vi "rsidr_core_global.vi"() -> ()   [LabVIEW 2015, in "Rohde&Schwarz CMXP GPRF.lvlib"] (continued)
"Read Callback"="", "Write Callback"="", "Supported Models"="", "Instrument Options"="", "Flags"=0, "Help"=""}, {"Level"=3, "Class Only"=FALSE, "Identifier"="RSCMXPGPRF_ATTR_GENERATOR_OUTPUT_CONNECTOR", "Descriptive Name"="Generator Output Connector", "Data Type"=0, "Command"="ROUT:GPRF:GEN{instance}:RFS:CONN", "Access"=2, "Range Table"="rsCmxpGprf_rngOutputConnector", "Read Callback"="", "Write Callback"="", "Supported Models"="", "Instrument Options"="", "Flags"=0, "Help"="Selects the output connector for the RF generator signal.\n\nAvailable Repeated Capabilities:\ninstance: i0, i1, i2, i3, i4, i5, i6, i7, i8, i9, i10, i11, i12, i13, i14, i15, i16, i17, i18, i19, i20, i21, i22, i23, i24, i25, i26, i27, i28, i29, i30, i31, i32\r\n\nRemote-control command(s):\nROUTe:GPRF:GEN<i>:RFSettings:CONNector"}, {"Level"=3, "Class Only"=FALSE, "Identifier"="RSCMXPGPRF_ATTR_GENERATOR_EXTERNAL_ATTENUTATION", "Descriptive Name"="Generator External Attenutation", "Data Type"=1, "Command"="SOUR:GPRF:GEN{instance}:RFS:EATT", "Access"=2, "Range Table"="rsCmxpGprf_rngExtAtt", "Read Callback"="", "Write Callback"="", "Supported Models"="", "Instrument Options"="", "Flags"=0, "Help"="Defines an external attenuation (or gain, if the value is negative), to be applied to the selected RF output connector.\n\nAvailable Repeated Capabilities:\ninstance: i0, i1, i2, i3, i4, i5, i6, i7, i8, i9, i10, i11, i12, i13, i14, i15, i16, i17, i18, i19, i20, i21, i22, i23, i24, i25, i26, i27, i28, i29, i30, i31, i32\r\n\nRemote-control command(s):\nSOURce:GPRF:GEN<i>:RFSettings:EATTenuation"}, {"Level"=2, "Class Only"=TRUE, "Identifier"="", "Descriptive Name"="Constant Frequency", "Data Type"=0, "Command"="", "Access"=0, "Range Table"="", "Read Callback"="", "Write Callback"="", "Supported Models"="", "Instrument Options"="", "Flags"=0, "Help"=""}, {"Level"=3, "Class Only"=FALSE, "Identifier"="RSCMXPGPRF_ATTR_GENERATOR_FREQUENCY", "Descriptive Name"="Generator Frequency", "Data Type"=1, "Command"="SOUR:GPRF:GEN{instance}:RFS:FREQ", "Access"=2, "Range Table"="rsCmxpGprf_rngCenterFrequency", "Read Callback"="", "Write Callback"="", "Supported Models"="", "Instrument Options"="", "Flags"=0, "Help"="Selects the frequency of the RF generator (Generator Frequency). Some of the baseband modes (modulation types) modify the generator frequency.\n\nAvailable Repeated Capabilities:\ninstance: i0, i1, i2, i3, i4, i5, i6, i7, i8, i9, i10, i11, i12, i13, i14, i15, i16, i17, i18, i19, i20, i21, i22, i23, i24, i25, i26, i27, i28, i29, i30, i31, i32\r\n\nRemote-control command(s):\nSOURce:GPRF:GEN<i>:RFSettings:FREQuency"}, {"Level"=3, "Class Only"=FALSE, "Identifier"="RSCMXPGPRF_ATTR_GENERATOR_BASE_LEVEL", "Descriptive Name"="Generator Base Level", "Data Type"=1, "Command"="SOUR:GPRF:GEN{instance}:RFS:LEV", "Access"=2, "Range Table"="rsCmxpGprf_rngGeneratorLevel", "Read Callback"="", "Write Callback"="", "Supported Models"="", "Instrument Options"="", "Flags"=0, "Help"="Sets the base level (Level (RMS)) of the constant-frequency RF generator.\n\nAvailable Repeated Capabilities:\ninstance: i0, i1, i2, i3, i4, i5, i6, i7, i8, i9, i10, i11, i12, i13, i14, i15, i16, i17, i18, i19, i20, i21, i22, i23, i24, i25, i26, i27, i28, i29, i30, i31, i32\r\n\nRemote-control command(s):\nSOURce:GPRF:GEN<i>:RFSettings:LEVel"}, {"Level"=3, "Class Only"=FALSE, "Identifier"="RSCMXPGPRF_ATTR_GENERATOR_PEAK_ENVELOPE_POWER", "Descriptive Name"="Generator Peak Envelope Power", "Data Type"=1, "Command"="SOUR:GPRF:GEN{instance}:RFS:PEP?", "Access"=0, "Range Table"="", "Read Callback"="", "Write Callback"="", "Supported Models"="", "Instrument Options"="", "Flags"=0, "Help"="Queries the &apos;Peak Envelope Power&apos; for single and dual-tone signals.\n\nAvailable Repeated Capabilities:\ninstance: i0, i1, i2, i3, i4, i5, i6, i7, i8, i9, i10, i11, i12, i13, i14, i15, i16, i17, i18, i19, i20, i21, i22, i23, i24, i25, i26, i27, i28, i29, i30, i31, i32\r\n\nRemote-control command(s):\nSOURce:GPRF:GEN<i>:RFSettings:PEPower?"}, {"Level"=3, "Class Only"=FALSE, "Identifier"="RSCMXPGPRF_ATTR_GENERATOR_DIGITAL_GAIN", "Descriptive Name"="Generator Digital Gain", "Data Type"=1, "Command"="SOUR:GPRF:GEN{instance}:RFS:DGA", "Access"=2, "Range Table"="rsCmxpGprf_rngDigitalGain", "Read Callback"="", "Write Callback"="", "Supported Models"="", "Instrument Options"="", "Flags"=0, "Help"="Defines or the digital gain of the constant-frequency RF generator.\n\nAvailable Repeated Capabilities:\ninstance: i0, i1, i2, i3, i4, i5, i6, i7, i8, i9, i10, i11, i12, i13, i14, i15, i16, i17, i18, i19, i20, i21, i22, i23, i24, i25, i26, i27, i28, i29, i30, i31, i32\r\n\nRemote-control command(s):\nSOURce:GPRF:GEN<i>:RFSettings:DGAin"}, {"Level"=2, "Class Only"=TRUE, "Identifier"="", "Descriptive Name"="Baseband", "Data Type"=0, "Command"="", "Access"=0, "Range Table"="", "Read Callback"="", "Write Callback"="", "Supported Models"="", "Instrument Options"="", "Flags"=0, "Help"=""}, {"Level"=3, "Class Only"=FALSE, "Identifier"="RSCMXPGPRF_ATTR_BASEBAND_MODE", "Descriptive Name"="Baseband Mode", "Data Type"=0, "Command"="SOUR:GPRF:GEN{instance}:BBM", "Access"=2, "Range Table"="rsCmxpGprf_rngBasebandMode", "Read Callback"="", "Write Callback"="", "Supported Models"="", "Instrument Options"="", "Flags"=0, "Help"="Selects the baseband mode for the generator signal.\n\nAvailable Repeated Capabilities:\ninstance: i0, i1, i2, i3, i4, i5, i6, i7, i8, i9, i10, i11, i12, i13, i14, i15, i16, i17, i18, i19, i20, i21, i22, i23, i24, i25, i26, i27, i28, i29, i30, i31, i32\r\n\nRemote-control command(s):\nSOURce:GPRF:GEN<i>:BBMode"}, {"Level"=3, "Class Only"=FALSE, "Identifier"="RSCMXPGPRF_ATTR_DUAL_TONE_RATIO", "Descriptive Name"="Dual Tone Ratio", "Data Type"=1, "Command"="SOUR:GPRF:GEN{instance}:DTON:RAT", "Access"=2, "Range Table"="rsCmxpGprf_rngDtoneRatio", "Read Callback"="", "Write Callback"="", "Supported Models"="", "Instrument Options"="", "Flags"=0, "Help"="Sets dual tone ratio.\n\nAvailable Repeated Capabilities:\ninstance: i0, i1, i2, i3, i4, i5, i6, i7, i8, i9, i10, i11, i12, i13, i14, i15, i16, i17, i18, i19, i20, i21, i22, i23, i24, i25, i26, i27, i28, i29, i30, i31, i32\r\n\nRemote-control command(s):\nSOURce:GPRF:GEN<i>:DTONe:RATio"}, {"Level"=3, "Class Only"=TRUE, "Identifier"="", "Descriptive Name"="Source", "Data Type"=0, "Command"="", "Access"=0, "Range Table"="", "Read Callback"="", "Write Callback"="", "Supported Models"="", "Instrument Options"="", "Flags"=0, "Help"="Put a help here"}, {"Level"=4, "Class Only"=FALSE, "Identifier"="RSCMXPGPRF_ATTR_DUAL_TONE_FREQUENCY", "Descriptive Name"="Dual Tone Frequency", "Data Type"=1, "Command"="SOUR:GPRF:GEN{instance}:DTON:OFR{source}", "Access"=2, "Range Table"="rsCmxpGprf_rngDtoneFrequency", "Read Callback"="", "Write Callback"="", "Supported Models"="", "Instrument Options"="", "Flags"=0, "Help"="Sets dual tone frequency on selected source.\n\nAvailable Repeated Capabilities:\ninstance: i0, i1, i2, i3, i4, i5, i6, i7, i8, i9, i10, i11, i12, i13, i14, i15, i16, i17, i18, i19, i20, i21, i22, i23, i24, i25, i26, i27, i28, i29, i30, i31, i32\r\nsource: s1, s2\r\n\nRemote-control command(s):\nSOURce:GPRF:GEN<i>:DTONe:OFRequency<source>"}, {"Level"=4, "Class Only"=FALSE, "Identifier"="RSCMXPGPRF_ATTR_DUAL_TONE_LEVEL", "Descriptive Name"="Dual Tone Level", "Data Type"=1, "Command"="SOUR:GPRF:GEN{instance}:DTON:LEV{source}?", "Access"=0, "Range Table"="", "Read Callback"="", "Write Callback"="", "Supported Models"="", "Instrument Options"="", "Flags"=0, "Help"="Queries the output level of the source signal <source>. The output level is a function of the generator output level and the ratio.\n\nAvailable Repeated Capabilities:\ninstance: i0, i1, i2, i3, i4, i5, i6, i7, i8, i9, i10, i11, i12, i13, i14, i15, i16, i17, i18, i19, i20, i21, i22, i23, i24, i25, i26, i27, i28, i29, i30, i31, i32\r\nsource: s1, s2\r\n\nRemote-control command(s):\nSOURce:GPRF:GEN<i>:DTONe:LEVel<source>?"}, {"Level"=3, "Class Only"=TRUE, "Identifier"="", "Descriptive Name"="Trigger", "Data Type"=0, "Command"="", "Access"=0, "Range Table"="", "Read Callback"="", "Write Callback"="", "Supported Models"="", "Instrument Options"="", "Flags"=0, "Help"="Contains attributes for baseband trigger settings."}, {"Level"=4, "Class Only"=FALSE, "Identifier"="RSCMXPGPRF_ATTR_BASEBAND_TRIGGER_CATALOG_SOURCE", "Descriptive Name"="Baseband Trigger Catalog Source", "Data Type"=2, "Command"="TRIG:GPRF:GEN{instance}:CAT:SOUR?", "Access"=0, "Range Table"="", "Read Callback"="", "Write Callback"="", "Supported Models"="", "Instrument Options"="", "Flags"=0, "Help"="Lists all trigger source values that can be set using TRIGger:GPRF:GEN<i>[:ARB]:SOURce.\n\nAvailable Repeated Capabilities:\ninstance: i0, i1, i2, i3, i4, i5, i6, i7, i8, i9, i10, i11, i12, i13, i14, i15, i16, i17, i18, i19, i20, i21, i22, i23, i24, i25, i26, i27, i28, i29, i30, i31, i32\r\n\nRemote-control command(s):\nTRIGger:GPRF:GEN<i>[:ARB]:CATalog:SOURce?"}, {"Level"=4, "Class Only"=FALSE, "Identifier"="RSCMXPGPRF_ATTR_BASEBAND_TRIGGER_SOURCE", "Descriptive Name"="Baseband Trigger Source", "Data Type"=2, "Command"="TRIG:GPRF:GEN{instance}:SOUR", "Access"=2, "Range Table"="", "Read Callback"="", "Write Callback"="", "Supported Models"="", "Instrument Options"="", "Flags"=0, "Help"="Selects the source of the trigger events. The supported values depend on the installed options. You can query a list of all supported values via TRIGger:GPRF:GEN<i>[:ARB]:CATalog:SOURce?.\n\nAvailable Repeated Capabilities:\ninstance: i0, i1, i2, i3, i4, i5, i6, i7, i8, i9, i10, i11, i12, i13, i14, i15, i16, i17, i18, i19, i20, i21, i22, i23, i24, i25, i26, i27, i28, i29, i30, i31, i32\r\n\nRemote-control command(s):\nTRIGger:GPRF:GEN<i>[:ARB]:SOURce"}, {"Level"=4, "Class Only"=FALSE, "Identifier"="RSCMXPGPRF_ATTR_BASEBAND_TRIGGER_DELAY", "Descriptive Name"="Baseband Trigger Delay", "Data Type"=1, "Command"="TRIG:GPRF:GEN{instance}:DEL", "Access"=2, "Range Table"="rsCmxpGprf_rngBasebandTriggerDelay", "Read Callback"="", "Write Callback"="", "Supported Models"="", "Instrument Options"="", "Flags"=0, "Help"="Sets the trigger delay.\n\nAvailable Repeated Capabilities:\ninstance: i0, i1, i2, i3, i4, i5, i6, i7, i8, i9, i10, i11, i12, i13, i14, i15, i16, i17, i18, i19, i20, i21, i22, i23, i24, i25, i26, i27, i28, i29, i30, i31, i32\r\n\nRemote-control command(s):\nTRIGger:GPRF:GEN<i>[:ARB]:DELay"}, {"Level"=4, "Class Only"=FALSE, "Identifier"="RSCMXPGPRF_ATTR_BASEBAND_TRIGGER_TIMEOUT_ENABLED", "Descriptive Name"="Baseband Trigger Timeout Enabled", "Data Type"=3, "Command"="TRIG:GPRF:GEN{instance}:TOUT", "Access"=2, "Range Table"="", "Read Callback"="", "Write Callback"="", "Supported Models"="", "Instrument Options"="", "Flags"=0, "Help"="Sets a time after which the started generator must have received a trigger event.\n\nAvailable Repeated Capabilities:\ninstance: i0, i1, i2, i3, i4, i5, i6, i7, i8, i9, i10, i11, i12, i13, i14, i15, i16, i17, i18, i19, i20, i21, i22, i23, i24, i25, i26, i27, i28, i29, i30, i31, i32\r\n\nRemote-control command(s):\nTRIGger:GPRF:GEN<i>:TOUT"}, {"Level"=4, "Class Only"=FALSE, "Identifier"="RSCMXPGPRF_ATTR_BASEBAND_TRIGGER_TIMEOUT", "Descriptive Name"="Baseband Trigger Timeout", "Data Type"=1, "Command"="TRIG:GPRF:GEN{instance}:TOUT", "Access"=2, "Range Table"="rsCmxpGprf_rngBasebandTriggerTimeout", "Read Callback"="", "Write Callback"="", "Supported Models"="", "Instrument Options"="", "Flags"=0, "Help"="Sets a time after which the started generator must have received a trigger event.\n\nAvailable Repeated Capabilities:\ninstance: i0, i1, i2, i3, i4, i5, i6, i7, i8, i9, i10, i11, i12, i13, i14, i15, i16, i17, i18, i19, i20, i21, i22, i23, i24, i25, i26, i27, i28, i29, i30, i31, i32\r\n\nRemote-control command(s):\nTRIGger:GPRF:GEN<i>:TOUT"}, {"Level"=2, "Class Only"=TRUE, "Identifier"="", "Descriptive Name"="ARB", "Data Type"=0, "Command"="", "Access"=0, "Range Table"="", "Read Callback"="", "Write Callback"="", "Supported Models"="", "Instrument Options"="", "Flags"=0, "Help"="This class configures the ARB system."}, {"Level"=3, "Class Only"=FALSE, "Identifier"="RSCMXPGPRF_ATTR_ARB_FILE", "Descriptive Name"="ARB File", "Data Type"=2, "Command"="SOUR:GPRF:GEN{instance}:ARB:FILE", "Access"=2, "Range Table"="", "Read Callback"="", "Write Callback"="", "Supported Models"="", "Instrument Options"="", "Flags"=0, "Help"="Selects a waveform file, to be used for the arbitrary waveform generator.\n\nAvailable Repeated Capabilities:\ninstance: i0, i1, i2, i3, i4, i5, i6, i7, i8, i9, i10, i11, i12, i13, i14, i15, i16, i17, i18, i19, i20, i21, i22, i23, i24, i25, i26, i27, i28, i29, i30, i31, i32\r\n\nRemote-control command(s):\nSOURce:GPRF:GEN<i>:ARB:FILE"}, {"Level"=3, "Class Only"=FALSE, "Identifier"="RSCMXPGPRF_ATTR_ARB_GET_FILE_ABS_PATH", "Descriptive Name"="ARB Get File With Abs Path", "Data Type"=2, "Command"="SOUR:GPRF:GEN{instance}:ARB:FILE?", "Access"=0, "Range Table"="", "Read Callback"="", "Write Callback"="", "Supported Models"="", "Instrument Options"="", "Flags"=0, "Help"="Returns the absolute path of selected waveform file.\n\nAvailable Repeated Capabilities:\ninstance: i0, i1, i2, i3, i4, i5, i6, i7, i8, i9, i10, i11, i12, i13, i14, i15, i16, i17, i18, i19, i20, i21, i22, i23, i24, i25, i26, i27, i28, i29, i30, i31, i32\r\n\nRemote-control command(s):\nSOURce:GPRF:GEN<i>:ARB:FILE? ABSP"}, {"Level"=3, "Class Only"=FALSE, "Identifier"="RSCMXPGPRF_ATTR_ARB_FILE_DATE", "Descriptive Name"="ARB File Date", "Data Type"=2, "Command"="SOUR:GPRF:GEN{instance}:ARB:FILE:DATE?", "Access"=0, "Range Table"="", "Read Callback"="", "Write Callback"="", "Supported Models"="", "Instrument Options"="", "Flags"=0, "Help"="Queries the date of the loaded waveform file.\n\nAvailable Repeated Capabilities:\ninstance: i0, i1, i2, i3, i4, i5, i6, i7, i8, i9, i10, i11, i12, i13, i14, i15, i16, i17, i18, i19, i20, i21, i22, i23, i24, i25, i26, i27, i28, i29, i30, i31, i32\r\n\nRemote-control command(s):\nSOURce:GPRF:GEN<i>:ARB:FILE:DATE?"}, {"Level"=3, "Class Only"=FALSE, "Identifier"="RSCMXPGPRF_ATTR_ARB_FILE_CLOCK_RATE", "Descriptive Name"="ARB File Clock Rate", "Data Type"=0, "Command"="SOUR:GPRF:GEN{instance}:ARB:CRAT?", "Access"=0, "Range Table"="", "Read Callback"="", "Write Callback"="", "Supported Models"="", "Instrument Options"="", "Flags"=0, "Help"="Queries the clock rate of the loaded waveform file. The clock rates of waveform file created with R&S WinIQSIM2 are compatible with the R&S CMW.\n\nAvailable Repeated Capabilities:\ninstance: i0, i1, i2, i3, i4, i5, i6, i7, i8, i9, i10, i11, i12, i13, i14, i15, i16, i17, i18, i19, i20, i21, i22, i23, i24, i25, i26, i27, i28, i29, i30, i31, i32\r\n\nRemote-control command(s):\nSOURce:GPRF:GEN<i>:ARB:CRATe?"}, {"Level"=3, "Class Only"=FALSE, "Identifier"="RSCMXPGPRF_ATTR_ARB_FILE_SAMPLES", "Descriptive Name"="ARB File Samples", "Data Type"=0, "Command"="SOUR:GPRF:GEN{instance}:ARB:SAMP?", "Access"=0, "Range Table"="", "Read Callback"="", "Write Callback"="", "Supported Models"="", "Instrument Options"="", "Flags"=0, "Help"="Queries the number of samples in the loaded waveform file.\n\nAvailable Repeated Capabilities:\ninstance: i0, i1, i2, i3, i4, i5, i6, i7, i8, i9, i10, i11, i12, i13, i14, i15, i16, i17, i18, i19, i20, i21, i22, i23, i24, i25, i26, i27, i28, i29, i30, i31, i32\r\n\nRemote-control command(s):\nSOURce:GPRF:GEN<i>:ARB:SAMPles?"}, {"Level"=3, "Class Only"=FALSE, "Identifier"="RSCMXPGPRF_ATTR_ARB_FILE_LEVEL_OFFSET", "Descriptive Name"="ARB File Level Offset", "Data Type"=1, "Command"="SOUR:GPRF:GEN{instance}:ARB:LOFF?", "Access"=0, "Range Table"="", "Read Callback"="", "Write Callback"="", "Supported Models"="", "Instrument Options"="", "Flags"=0, "Help"="Queries the level offset of the loaded waveform file.\n\nAvailable Repeated Capabilities:\ninstance: i0, i1, i2, i3, i4, i5, i6, i7, i8, i9, i10, i11, i12, i13, i14, i15, i16, i17, i18, i19, i20, i21, i22, i23, i24, i25, i26, i27, i28, i29, i30, i31, i32\r\n\nRemote-control command(s):\nSOURce:GPRF:GEN<i>:ARB:LOFFset?"}, {"Level"=3, "Class Only"=FALSE, "Identifier"="RSCMXPGPRF_ATTR_ARB_FILE_PEAK_OFFSET", "Descriptive Name"="ARB File Peak Offset", "Data Type"=1, "Command"="SOUR:GPRF:GEN{instance}:ARB:POFF?", "Access"=0, "Range Table"="", "Read Callback"="", "Write Callback"="", "Supported Models"="", "Instrument Options"="", "Flags"=0, "Help"="Queries the peak offset of the loaded waveform file.\n\nAvailable Repeated Capabilities:\ninstance: i0, i1, i2, i3, i4, i5, i6, i7, i8, i9, i10, i11, i12, i13, i14, i15, i16, i17, i18, i19, i20, i21, i22, i23, i24, i25, i26, i27, i28, i29, i30, i31, i32\r\n\nRemote-control command(s):\nSOURce:GPRF:GEN<i>:ARB:POFFset?"}, {"Level"=3, "Class Only"=FALSE, "Identifier"="RSCMXPGPRF_ATTR_ARB_FILE_CRC_PROTECTION", "Descriptive Name"="ARB File CRC Protection", "Data Type"=0, "Command"="SOUR:GPRF:GEN{instance}:ARB:CRCP?", "Access"=0, "Range Table"="rsCmxpGprf_rngARBFileCRCProtection", "Read Callback"="", "Write Callback"="", "Supported Models"="", "Instrument Options"="", "Flags"=0, "Help"="Queries whether the loaded ARB file contains a CRC checksum, which could be used for an integrity check\n\nAvailable Repeated Capabilities:\ninstance: i0, i1, i2, i3, i4, i5, i6, i7, i8, i9, i10, i11, i12, i13, i14, i15, i16, i17, i18, i19, i20, i21, i22, i23, i24, i25, i26, i27, i28, i29, i30, i31, i32\r\n\nRemote-control command(s):\nSOURce:GPRF:GEN<i>:ARB:CRCProtect?"}, {"Level"=3, "Class Only"=FALSE, "Identifier"="RSCMXPGPRF_ATTR_ARB_FILE_VERSION", "Descriptive Name"="ARB File Version", "Data Type"=2, "Command"="SOUR:GPRF:GEN{instance}:ARB:FILE:VERS?", "Access"=0, "Range Table"="", "Read Callback"="", "Write Callback"="", "Supported Models"="", "Instrument Options"="", "Flags"=0, "Help"="Queries the version of the loaded waveform file.\n\nAvailable Repeated Capabilities:\ninstance: i0, i1, i2, i3, i4, i5, i6, i7, i8, i9, i10, i11, i12, i13, i14, i15, i16, i17, i18, i19, i20, i21, i22, i23, i24, i25, i26, i27, i28, i29, i30, i31, i32\r\n\nRemote-control command(s):\nSOURce:GPRF:GEN<i>:ARB:FILE:VERSion?"}, {"Level"=3, "Class Only"=FALSE, "Identifier"="RSCMXPGPRF_ATTR_ARB_FILE_OPTION", "Descriptive Name"="ARB File Option", "Data Type"=2, "Command"="SOUR:GPRF:GEN{instance}:ARB:FILE:OPT?", "Access"=0, "Range Table"="", "Read Callback"="", "Write Callback"="", "Supported Models"="", "Instrument Options"="", "Flags"=0, "Help"="Queries the R&S CMW-KV and R&S CMW-KW-options that are required to process the loaded ARB file with the arbitrary RF generator.\n\nAvailable Repeated Capabilities:\ninstance: i0, i1, i2, i3, i4, i5, i6, i7, i8, i9, i10, i11, i12, i13, i14, i15, i16, i17, i18, i19, i20, i21, i22, i23, i24, i25, i26, i27, i28, i29, i30, i31, i32\r\n\nRemote-control command(s):\nSOURce:GPRF:GEN<i>:ARB:FILE:OPTion?"}, {"Level"=3, "Class Only"=FALSE, "Identifier"="RSCMXPGPRF_ATTR_ARB_FILE_SAMPLES_SUBRANGE", "Descriptive Name"="ARB File Samples Subrange", "Data Type"=6, "Command"="SOUR:GPRF:GEN{instance}:ARB:SAMP:RANG", "Access"=2, "Range Table"="", "Read Callback"="", "Write Callback"="", "Supported Models"="", "Instrument Options"="", "Flags"=0, "Help"="Defines the range of samples in the loaded ARB file that are processed.\n\nParameters: <Range>[, <Start>, <Stop>]\n- <Range> FULL | SUB\n- <Start> integer\n- <Stop> integer\n\nAvailable Repeated Capabilities:\ninstance: i0, i1, i2, i3, i4, i5, i6, i7, i8, i9, i10, i11, i12, i13, i14, i15, i16, i17, i18, i19, i20, i21, i22, i23, i24, i25, i26, i27, i28, i29, i30, i31, i32\r\n\nRemote-control command(s):\nSOURce:GPRF:GEN<i>:ARB:SAMPles:RANGe"}, {"Level"=2, "Class Only"=TRUE, "Identifier"="", "Descriptive Name"="Sequencer", "Data Type"=0, "Command"="", "Access"=0, "Range Table"="", "Read Callback"="", "Write Callback"="", "Supported Models"="", "Instrument Options"="", "Flags"=0, "Help"="The sequencer mode is in the current software version only supported by the R&S CMW100.\nThis operation mode is much easier to use than the older generator mode. It supports a wide bandwidth of signal types, from a simple continuous CW signal to a complex sequence of different signals involving several ARB waveform files.\nThe signals to be generated are configured via the sequencer list. Each list entry defines a signal, including RF settings like frequency and level, and baseband settings."}, {"Level"=3, "Class Only"=FALSE, "Identifier"="RSCMXPGPRF_ATTR_SEQUENCE_REPETITION", "Descriptive Name"="Sequence Repetition", "Data Type"=0, "Command"="SOUR:GPRF:GEN{instance}:SEQ:REP", "Access"=2, "Range Table"="rsCmxpGprf_rngRepMode", "Read Callback"="", "Write Callback"="", "Supported Models"="", "Instrument Options"="", "Flags"=0, "Help"="Defines how often the sequencer list is processed.\n\nAvailable Repeated Capabilities:\ninstance: i0, i1, i2, i3, i4, i5, i6, i7, i8, i9, i10, i11, i12, i13, i14, i15, i16, i17, i18, i19, i20, i21, i22, i23, i24, i25, i26, i27, i28, i29, i30, i31, i32\r\n\nRemote-control command(s):\nSOURce:GPRF:GEN<i>:SEQuencer:REPetition"}, {"Level"=3, "Class Only"=FALSE, "Identifier"="RSCMXPGPRF_ATTR_SEQUENCE_REPETITION_COUNT", "Descriptive Name"="Sequence Repetition Count", "Data Type"=0, "Command"="SOUR:GPRF:GEN{instance}:SEQ:NREP", "Access"=2, "Range Table"="rsCmxpGprf_rngSequenceRepetitionCount", "Read Callback"="", "Write Callback"="", "Supported Models"="", "Instrument Options"="", "Flags"=0, "Help"="Defines how often the sequencer list is processed in SINGle repetition mode.\n\nAvailable Repeated Capabilities:\ninstance: i0, i1, i2, i3, i4, i5, i6, i7, i8, i9, i10, i11, i12, i13, i14, i15, i16, i17, i18, i19, i20, i21, i22, i23, i24, i25, i26, i27, i28, i29, i30, i31, i32\r\n\nRemote-control command(s):\nSOURce:GPRF:GEN<i>:SEQuencer:NREPetition"}, {"Level"=3, "Class Only"=FALSE, "Identifier"="RSCMXPGPRF_ATTR_SEQUENCE_COMPLETED_REPETITIONS", "Descriptive Name"="Sequence Completed Repetitions", "Data Type"=0, "Command"="SOUR:GPRF:GEN{instance}:SEQ:RCO?", "Access"=0, "Range Table"="", "Read Callback"="", "Write Callback"="", "Supported Models"="", "Instrument Options"="", "Flags"=0, "Help"="Queries the number of completed repetitions of the sequencer list, for repetition mode SINGle.\n\nAvailable Repeated Capabilities:\ninstance: i0, i1, i2, i3, i4, i5, i6, i7, i8, i9, i10, i11, i12, i13, i14, i15, i16, i17, i18, i19, i20, i21, i22, i23, i24, i25, i26, i27, i28, i29, i30, i31, i32\r\n\nRemote-control command(s):\nSOURce:GPRF:GEN<i>:SEQuencer:RCOunt?"}, {"Level"=3, "Class Only"=FALSE, "Identifier"="RSCMXPGPRF_ATTR_SEQUENCER_CONNECTOR", "Descriptive Name"="Sequencer Connector", "Data Type"=2, "Command"="ROUT:GPRF:GEN{instance}:SPAT", "Access"=2, "Range Table"="", "Read Callback"="", "Write Callback"="", "Supported Models"="", "Instrument Options"="", "Flags"=0, "Help"="Selects the output connector for the generated signal.\n\nAvailable Repeated Capabilities:\ninstance: i0, i1, i2, i3, i4, i5, i6, i7, i8, i9, i10, i11, i12, i13, i14, i15, i16, i17, i18, i19, i20, i21, i22, i23, i24, i25, i26, i27, i28, i29, i30, i31, i32\r\n\nRemote-control command(s):\nROUTe:GPRF:GEN<i>:SPATh"}, {"Level"=3, "Class Only"=FALSE, "Identifier"="RSCMXPGPRF_ATTR_SEQUENCER_CONNECTION_AVAILABLE_SIGNAL_PATHS", "Descriptive Name"="Sequencer Connection Available Signal Paths", "Data Type"=2, "Command"="CAT:GPRF:GEN{instance}:SPAT?", "Access"=0, "Range Table"="", "Read Callback"="", "Write Callback"="", "Supported Models"="", "Instrument Options"="", "Flags"=0, "Help"="Returns the names of the available signal paths.\n\nAvailable Repeated Capabilities:\ninstance: i0, i1, i2, i3, i4, i5, i6, i7, i8, i9, i10, i11, i12, i13, i14, i15, i16, i17, i18, i19, i20, i21, i22, i23, i24, i25, i26, i27, i28, i29, i30, i31, i32\r\n\nRemote-control command(s):\nCATalog:GPRF:GEN<i>:SPATh<stream>?"}, {"Level"=3, "Class Only"=FALSE, "Identifier"="RSCMXPGPRF_ATTR_SEQUENCER_ARB_TDD_MODE", "Descriptive Name"="Sequencer ARB TDD Mode", "Data Type"=3, "Command"="SOUR:GPRF:GEN{instance}:SEQ:TDD:MODE", "Access"=2, "Range Table"="", "Read Callback"="", "Write Callback"="", "Supported Models"="", "Instrument Options"="", "Flags"=0, "Help"="Enables or disables the TDD mode for a signal output path with a remote radio head (RRH).\n\nAvailable Repeated Capabilities:\ninstance: i0, i1, i2, i3, i4, i5, i6, i7, i8, i9, i10, i11, i12, i13, i14, i15, i16, i17, i18, i19, i20, i21, i22, i23, i24, i25, i26, i27, i28, i29, i30, i31, i32\r\n\nRemote-control command(s):\nSOURce:GPRF:GEN<i>:SEQuencer:TDD:MODE"}, {"Level"=3, "Class Only"=FALSE, "Identifier"="RSCMXPGPRF_ATTR_SEQUENCER_STATUS_ALL", "Descriptive Name"="Sequencer Status All", "Data Type"=6, "Command"="SOUR:GPRF:GEN{instance}:SEQ:STAT:ALL?", "Access"=0, "Range Table"="", "Read Callback"="", "Write Callback"="", "Supported Models"="", "Instrument Options"="", "Flags"=0, "Help"="Queries the main measurement state and the measurement substates. Both measurement substates are relevant for running measurements only.\n\nAvailable Repeated Capabilities:\ninstance: i0, i1, i2, i3, i4, i5, i6, i7, i8, i9, i10, i11, i12, i13, i14, i15, i16, i17, i18, i19, i20, i21, i22, i23, i24, i25, i26, i27, i28, i29, i30, i31, i32\r\n\nRemote-control command(s):\nSOURce:GPRF:GEN<i>:SEQuencer:STATe:ALL?"}, {"Level"=3, "Class Only"=TRUE, "Identifier"="", "Descriptive Name"="Control", "Data Type"=0, "Command"="", "Access"=0, "Range Table"="", "Read Callback"="", "Write Callback"="", "Supported Models"="", "Instrument Options"="", "Flags"=0, "Help"="The following attributes control the sequencer state, retrieve status information and report problems."}, {"Level"=4, "Class Only"=FALSE, "Identifier"="RSCMXPGPRF_ATTR_SEQUENCER_STATE", "Descriptive Name"="Sequencer State", "Data Type"=3, "Command"="SOUR:GPRF:GEN{instance}:SEQ:STAT", "Access"=2, "Range Table"="", "Read Callback"="", "Write Callback"="", "Supported Models"="", "Instrument Options"="", "Flags"=0, "Help"="Turns the sequencer on or off.\n\nAvailable Repeated Capabilities:\ninstance: i0, i1, i2, i3, i4, i5, i6, i7, i8, i9, i10, i11, i12, i13, i14, i15, i16, i17, i18, i19, i20, i21, i22, i23, i24, i25, i26, i27, i28, i29, i30, i31, i32\r\n\nRemote-control command(s):\nSOURce:GPRF:GEN<i>:SEQuencer:STATe"}, {"Level"=4, "Class Only"=FALSE, "Identifier"="RSCMXPGPRF_ATTR_QUERY_SEQUENCER_STATE", "Descriptive Name"="Query Sequencer State", "Data Type"=0, "Command"="SOUR:GPRF:GEN{instance}:SEQ:STAT?", "Access"=0, "Range Table"="rsCmxpGprf_rngGeneratorState", "Read Callback"="", "Write Callback"="", "Supported Models"="", "Instrument Options"="", "Flags"=0, "Help"="Queries sequencer state.\n\nAvailable Repeated Capabilities:\ninstance: i0, i1, i2, i3, i4, i5, i6, i7, i8, i9, i10, i11, i12, i13, i14, i15, i16, i17, i18, i19, i20, i21, i22, i23, i24, i25, i26, i27, i28, i29, i30, i31, i32\r\n\nRemote-control command(s):\nSOURce:GPRF:GEN<i>:SEQuencer:STATe?"}, {"Level"=4, "Class Only"=FALSE, "Identifier"="RSCMXPGPRF_ATTR_SEQUENCER_SIGNAL", "Descriptive Name"="Sequencer Signal", "Data Type"=3, "Command"="SOUR:GPRF:GEN{instance}:SEQ:SIGN?", "Access"=0, "Range Table"="", "Read Callback"="", "Write Callback"="", "Supported Models"="", "Instrument Options"="", "Flags"=0, "Help"="Queries whether a signal is generated or not.\n\nAvailable Repeated Capabilities:\ninstance: i0, i1, i2, i3, i4, i5, i6, i7, i8, i9, i10, i11, i12, i13, i14, i15, i16, i17, i18, i19, i20, i21, i22, i23, i24, i25, i26, i27, i28, i29, i30, i31, i32\r\n\nRemote-control command(s):\nSOURce:GPRF:GEN<i>:SEQuencer:SIGNal?"}, {"Level"=4, "Class Only"=FALSE, "Identifier"="RSCMXPGPRF_ATTR_SEQUENCER_INDEX", "Descriptive Name"="Sequencer Index", "Data Type"=0, "Command"="SOUR:GPRF:GEN{instance}:SEQ:CENT?", "Access"=0, "Range Table"="", "Read Callback"="", "Write Callback"="", "Supported Models"="", "Instrument Options"="", "Flags"=0, "Help"="Queries the index of the processed entry.\n\nAvailable Repeated Capabilities:\ninstance: i0, i1, i2, i3, i4, i5, i6, i7, i8, i9, i10, i11, i12, i13, i14, i15, i16, i17, i18, i19, i20, i21, i22, i23, i24, i25, i26, i27, i28, i29, i30, i31, i32\r\n\nRemote-control command(s):\nSOURce:GPRF:GEN<i>:SEQuencer:CENTry?"}, {"Level"=4, "Class Only"=FALSE, "Identifier"="RSCMXPGPRF_ATTR_SEQUENCER_USED_OPTIONS", "Descriptive Name"="Sequencer Used Options", "Data Type"=2, "Command"="SOUR:GPRF:GEN{instance}:SEQ:UOPT?", "Access"=0, "Range Table"="", "Read Callback"="", "Write Callback"="", "Supported Models"="", "Instrument Options"="", "Flags"=0, "Help"="Queries a list of the used software options.\n\nAvailable Repeated Capabilities:\ninstance: i0, i1, i2, i3, i4, i5, i6, i7, i8, i9, i10, i11, i12, i13, i14, i15, i16, i17, i18, i19, i20, i21, i22, i23, i24, i25, i26, i27, i28, i29, i30, i31, i32\r\n\nRemote-control command(s):\nSOURce:GPRF:GEN<i>:SEQuencer:UOPTions?"}, {"Level"=4, "Class Only"=FALSE, "Identifier"="RSCMXPGPRF_ATTR_SEQUENCER_RELIABILITY", "Descriptive Name"="Sequencer Reliability", "Data Type"=6, "Command"="SOUR:GPRF:GEN{instance}:SEQ:REL:ALL?", "Access"=0, "Range Table"="", "Read Callback"="", "Write Callback"="", "Supported Models"="", "Instrument Options"="", "Flags"=0, "Help"="Reports if and why there are problems generating the configured signal.\n\nAvailable Repeated Capabilities:\ninstance: i0, i1, i2, i3, i4, i5, i6, i7, i8, i9, i10, i11, i12, i13, i14, i15, i16, i17, i18, i19, i20, i21, i22, i23, i24, i25, i26, i27, i28, i29, i30, i31, i32\r\n\nRemote-control command(s):\nSOURce:GPRF:GEN<i>:SEQuencer:RELiability:ALL?"}, {"Level"=3, "Class Only"=TRUE, "Identifier"="", "Descriptive Name"="ARB File Pool", "Data Type"=0, "Command"="", "Access"=0, "Range Table"="", "Read Callback"="", "Write Callback"="", "Supported Models"="", "Instrument Options"="", "Flags"=0, "Help"="ARB file pool settings"}, {"Level"=4, "Class Only"=FALSE, "Identifier"="RSCMXPGPRF_ATTR_SEQUENCER_ADD_ARB_FILE", "Descriptive Name"="Sequencer Add ARB File", "Data Type"=2, "Command"="SOUR:GPRF:GEN{instance}:SEQ:APO:FILE", "Access"=1, "Range Table"="", "Read Callback"="", "Write Callback"="", "Supported Models"="", "Instrument Options"="", "Flags"=0, "Help"="Adds an ARB file to the ARB file pool.\n\nAvailable Repeated Capabilities:\ninstance: i0, i1, i2, i3, i4, i5, i6, i7, i8, i9, i10, i11, i12, i13, i14, i15, i16, i17, i18, i19, i20, i21, i22, i23, i24, i25, i26, i27, i28, i29, i30, i31, i32\r\n\nRemote-control command(s):\nSOURce:GPRF:GEN<i>:SEQuencer:APOol:FILE"}, {"Level"=4, "Class Only"=FALSE, "Identifier"="RSCMXPGPRF_ATTR_SEQUENCER_CLEAR_ARB_POOL", "Descriptive Name"="Sequencer Clear ARB Pool", "Data Type"=4, "Command"="SOUR:GPRF:GEN{instance}:SEQ:APO:CLE", "Access"=1, "Range Table"="", "Read Callback"="", "Write Callback"="", "Supported Models"="", "Instrument Options"="", "Flags"=0, "Help"="Removes all files from the ARB file pool.\n\nAvailable Repeated Capabilities:\ninstance: i0, i1, i2, i3, i4, i5, i6, i7, i8, i9, i10, i11, i12, i13, i14, i15, i16, i17, i18, i19, i20, i21, i22, i23, i24, i25, i26, i27, i28, i29, i30, i31, i32\r\n\nRemote-control command(s):\nSOURce:GPRF:GEN<i>:SEQuencer:APOol:CLEar"}, {"Level"=4, "Class Only"=FALSE, "Identifier"="RSCMXPGPRF_ATTR_SEQUENCER_REMOVE_ARB_FILES", "Descriptive Name"="Sequencer Remove ARB Files", "Data Type"=6, "Command"="SOUR:GPRF:GEN{instance}:SEQ:APO:REM", "Access"=1, "Range Table"="", "Read Callback"="", "Write Callback"="", "Supported Models"="", "Instrument Options"="", "Flags"=0, "Help"="Removes selected files from the ARB file pool.\n\nAvailable Repeated Capabilities:\ninstance: i0, i1, i2, i3, i4, i5, i6, i7, i8, i9, i10, i11, i12, i13, i14, i15, i16, i17, i18, i19, i20, i21, i22, i23, i24, i25, i26, i27, i28, i29, i30, i31, i32\r\n\nRemote-control command(s):\nSOURce:GPRF:GEN<i>:SEQuencer:APOol:REMove"}, {"Level"=4, "Class Only"=FALSE, "Identifier"="RSCMXPGPRF_ATTR_SEQUENCER_DOWNLOAD_TO_ARB_RAM", "Descriptive Name"="Sequencer Download To ARB RAM", "Data Type"=4, "Command"="SOUR:GPRF:GEN{instance}:SEQ:APO:DOWN", "Access"=1, "Range Table"="", "Read Callback"="", "Write Callback"="", "Supported Models"="", "Instrument Options"="", "Flags"=0, "Help"="Downloads the ARB files from the file pool to the ARB RAM.\n\nAvailable Repeated Capabilities:\ninstance: i0, i1, i2, i3, i4, i5, i6, i7, i8, i9, i10, i11, i12, i13, i14, i15, i16, i17, i18, i19, i20, i21, i22, i23, i24, i25, i26, i27, i28, i29, i30, i31, i32\r\n\nRemote-control command(s):\nSOURce:GPRF:GEN<i>:SEQuencer:APOol:DOWNload"}, {"Level"=4, "Class Only"=FALSE, "Identifier"="RSCMXPGPRF_ATTR_SEQUENCER_ARB_FILE_POOL_VALID", "Descriptive Name"="Sequencer ARB File Pool Valid", "Data Type"=0, "Command"="SOUR:GPRF:GEN{instance}:SEQ:APO:VAL?", "Access"=0, "Range Table"="rsCmxpGprf_rngNoYesNav", "Read Callback"="", "Write Callback"="", "Supported Models"="", "Instrument Options"="", "Flags"=0, "Help"="Queries whether the ARB file pool is valid.\n\nAvailable Repeated Capabilities:\ninstance: i0, i1, i2, i3, i4, i5, i6, i7, i8, i9, i10, i11, i12, i13, i14, i15, i16, i17, i18, i19, i20, i21, i22, i23, i24, i25, i26, i27, i28, i29, i30, i31, i32\r\n\nRemote-control command(s):\nSOURce:GPRF:GEN<i>:SEQuencer:APOol:VALid?"}, {"Level"=4, "Class Only"=FALSE, "Identifier"="RSCMXPGPRF_ATTR_SEQUENCER_ARB_FILE_POOL_DOWNLOADED", "Descriptive Name"="Sequencer ARB File Pool Downloaded", "Data Type"=0, "Command"="SOUR:GPRF:GEN{instance}:SEQ:APO:LOAD?", "Access"=0, "Range Table"="rsCmxpGprf_rngNoYesNav", "Read Callback"="", "Write Callback"="", "Supported Models"="", "Instrument Options"="", "Flags"=0, "Help"="Queries whether the ARB file pool is downloaded to the ARB RAM.\n\nAvailable Repeated Capabilities:\ninstance: i0, i1, i2, i3, i4, i5, i6, i7, i8, i9, i10, i11, i12, i13, i14, i15, i16, i17, i18, i19, i20, i21, i22, i23, i24, i25, i26, i27, i28, i29, i30, i31, i32\r\n\nRemote-control command(s):\nSOURce:GPRF:GEN<i>:SEQuencer:APOol:LOADed?"}, {"Level"=4, "Class Only"=FALSE, "Identifier"="RSCMXPGPRF_ATTR_SEQUENCER_ARB_RAM_REQUIRED", "Descriptive Name"="Sequencer ARB RAM Required", "Data Type"=0, "Command"="SOUR:GPRF:GEN{instance}:SEQ:APO:RREQ?", "Access"=0, "Range Table"="", "Read Callback"="", "Write Callback"="", "Supported Models"="", "Instrument Options"="", "Flags"=0, "Help"="Queries the amount of RAM in MBytes required by the ARB files in the pool.\n\nAvailable Repeated Capabilities:\ninstance: i0, i1, i2, i3, i4, i5, i6, i7, i8, i9, i10, i11, i12, i13, i14, i15, i16, i17, i18, i19, i20, i21, i22, i23, i24, i25, i26, i27, i28, i29, i30, i31, i32\r\n\nRemote-control command(s):\nSOURce:GPRF:GEN<i>:SEQuencer:APOol:RREQuired?"}, {"Level"=4, "Class Only"=FALSE, "Identifier"="RSCMXPGPRF_ATTR_SEQUENCER_RAM_TOTAL", "Descriptive Name"="Sequencer RAM Total", "Data Type"=0, "Command"="SOUR:GPRF:GEN{instance}:SEQ:APO:RTOT?", "Access"=0, "Range Table"="", "Read Callback"="", "Write Callback"="", "Supported Models"="", "Instrument Options"="", "Flags"=0, "Help"="Queries the amount of RAM in MBytes available for ARB files.\n\nAvailable Repeated Capabilities:\ninstance: i0, i1, i2, i3, i4, i5, i6, i7, i8, i9, i10, i11, i12, i13, i14, i15, i16, i17, i18, i19, i20, i21, i22, i23, i24, i25, i26, i27, i28, i29, i30, i31, i32\r\n\nRemote-control command(s):\nSOURce:GPRF:GEN<i>:SEQuencer:APOol:RTOTal?"}, {"Level"=4, "Class Only"=FALSE, "Identifier"="RSCMXPGPRF_ATTR_SEQUENCER_MAXIMUM_INDEX", "Descriptive Name"="Sequencer Maximum Index", "Data Type"=0, "Command"="SOUR:GPRF:GEN{instance}:SEQ:APO:MIND?", "Access"=0, "Range Table"="", "Read Callback"="", "Write Callback"="", "Supported Models"="", "Instrument Options"="", "Flags"=0, "Help"="Queries the highest index of the ARB file pool. The pool contains files with the indices 0 to <MaximumIndex>.\n\nAvailable Repeated Capabilities:\ninstance: i0, i1, i2, i3, i4, i5, i6, i7, i8, i9, i10, i11, i12, i13, i14, i15, i16, i17, i18, i19, i20, i21, i22, i23, i24, i25, i26, i27, i28, i29, i30, i31, i32\r\n\nRemote-control command(s):\nSOURce:GPRF:GEN<i>:SEQuencer:APOol:MINDex?"}, {"Level"=4, "Class Only"=FALSE, "Identifier"="RSCMXPGPRF_ATTR_HIDDEN_SEQUENCER_ARB_FILE_NAME", "Descriptive Name"="Sequencer ARB File Name", "Data Type"=2, "Command"="SOUR:GPRF:GEN{instance}:SEQ:APO:WAV?", "Access"=0, "Range Table"="", "Read Callback"="", "Write Callback"="", "Supported Models"="", "Instrument Options"="", "Flags"=8, "Help"="Queries the name of the ARB file with the specified <Index>.\n\nAvailable Repeated Capabilities:\ninstance: i0, i1, i2, i3, i4, i5, i6, i7, i8, i9, i10, i11, i12, i13, i14, i15, i16, i17, i18, i19, i20, i21, i22, i23, i24, i25, i26, i27, i28, i29, i30, i31, i32\r\n\nRemote-control command(s):\nSOURce:GPRF:GEN<i>:SEQuencer:APOol:WAVeform?"}, {"Level"=4, "Class Only"=FALSE, "Identifier"="RSCMXPGPRF_ATTR_SEQUENCER_ARB_FILE_ALL_NAMES", "Descriptive Name"="Sequencer 
